vi "rad_FilterTargets.vi"(10 "Target Types":string[](array[string]), 11 "Targets Information":T1[](array[typedef]) {"Primary NIC"."IP Address Request Mode" items=["Static"=1, "DHCP/Link-Local"=2, "Link-Local Only"=4, "DHCP Only"=8]}) -> (1 "Filtered Targets":i32[](array[numeric]), 3 "Targets Information":T1[](array[typedef]) {"Primary NIC"."IP Address Request Mode" items=["Static"=1, "DHCP/Link-Local"=2, "Link-Local Only"=4, "DHCP Only"=8]})   [LabVIEW 2016]
uses:
  TypeDefs/rad_Target Information.ctl
  TypeDefs/rad_Target Network Settings.ctl
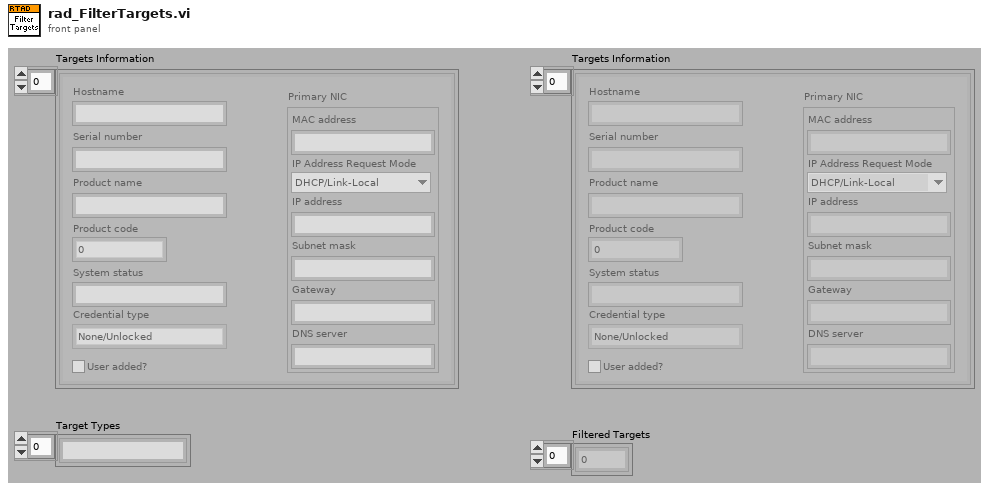
[diagram p1: front panel]
types:
  T1 = typedef "rad_Target Information.ctl" = cluster{"Hostname":string, "Serial number":string, "Product name":string, "Product code":i32, "System status":string, "Credential type":enum16{"None/Unlocked", "FTP Password", "NIAuth Credentials"}, "User added?":bool, "Primary NIC":T2}
  T2 = typedef "rad_Target Network Settings.ctl" = cluster{"MAC address":string, "IP Address Request Mode":i32, "IP address":string, "Subnet mask":string, "Gateway":string, "DNS server":string}
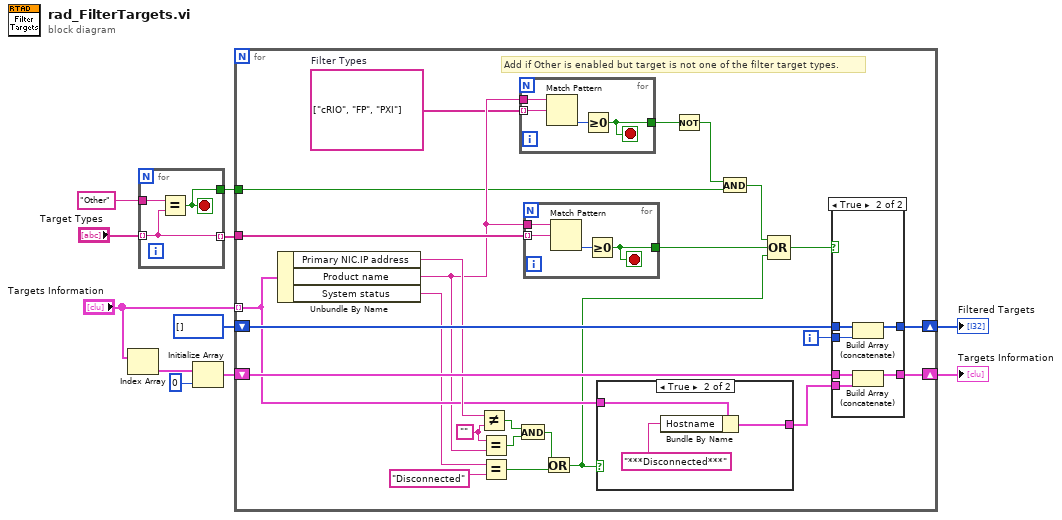
[diagram p0: block diagram]
diagram:
  n1 = Index Array(array="Targets Information") -> (element=w10:T1)  [unwired: 1 in]
  n2 = for {
    tunnel: "Target Types" -> [w13] mode=indexing
    tunnel: [w13] -> w3 mode=indexing
    tunnel: "Other" ("y") -> [w12]
    tunnel: [w14] -> w1
    stop <- w14 stop-if-true
    n3 = Equal?(x=w12, y=w13) -> (x = y?=w14:bool)
  }
  n4 = Initialize Array(w10, 0 ("dimension size")) -> (w9:T1[])
  n5 = for {
    shift-right: [w38] -> w7
    shift-left: w9 -> [w39]
    tunnel: "Targets Information" -> [w28] mode=indexing
    tunnel: w3 -> [w37]
    shift-right: [w35] -> w5
    shift-left: i32[] [] -> [w34]
    tunnel: w1 -> [w16]
    i -> [w36]
    w19 = string[] ["cRIO", "FP", "PXI"]  # Filter Types
    w32 = ""
    # "Add if Other is enabled but target is not one of the filter target types."
    n6 = Unbundle By Name(w28) -> ("Primary NIC.IP address"=w33:string, "Product name"=w20:string, "System status"=w26:string)
    n7 = Not Equal?(x=w33, y=w32) -> (x != y?=w31:bool)
    n8 = Equal?(x=w32, y=w20) -> (x = y?=w30:bool)
    n9 = Equal?(x=w26, y="Disconnected") -> (x = y?=w23:bool)
    n10 = And(x=w31, y=w30) -> (x .and. y?=w24:bool)
    n11 = for {
      tunnel: w20 -> [w43]
      tunnel: w19 -> [w42] mode=indexing
      tunnel: [w40] -> w18
      stop <- w40 stop-if-true
      n12 = Match Pattern(string=w43, regular expression=w42) -> (offset past match=w41:i32)  [unwired: 4 out]
      n13 = Greater Or Equal To 0?(x=w41) -> (x >= 0?=w40:bool)
    }
    n14 = for {
      tunnel: w20 -> [w51]
      tunnel: w37 -> [w50] mode=indexing
      tunnel: [w48] -> w21
      stop <- w48 stop-if-true
      n15 = Match Pattern(string=w51, regular expression=w50) -> (offset past match=w49:i32)  [unwired: 4 out]
      n16 = Greater Or Equal To 0?(x=w49) -> (x >= 0?=w48:bool)
    }
    n17 = Or(x=w24, y=w23) -> (x .or. y?=w22:bool)
    n18 = case shown="True" w22 {
      tunnel: w28 -> [w44 w47]
      tunnel: [w44 w45] -> w27
      frame False {
      }
      frame True {
        n19 = Bundle By Name(cluster=w47, "Hostname"="***Disconnected***" ("IP settings.DNS name")) -> (w45:T1)
      }
    }
    n20 = Not(x=w18) -> (.not. x?=w17:bool)
    n21 = And(x=w17, y=w16) -> (x .and. y?=w15:bool)
    n22 = Compound Arithmetic op=OR(w15, w21, w22) -> (w29:bool)
    n23 = case shown="True" w29 {
      tunnel: w39 -> [w53 w59]
      tunnel: [w53 w57] -> w38
      tunnel: w27 -> [_ w58]
      tunnel: w36 -> [_ w56]
      tunnel: [w52 w55] -> w35
      tunnel: w34 -> [w52 w54]
      frame False {
      }
      frame True {
        n24 = Build Array (concatenate)(w54, w56) -> (w55:i32[])
        n25 = Build Array (concatenate)(w59, w58) -> (w57:T1[])
      }
    }
  }
  "Targets Information" <- w7
  "Filtered Targets" <- w5
